vi "Add Keywords Popup Dialog.vi"(8 "error in (no error)":errorcluster, 11 "Keywords In":string[](array[string])) -> (0 "error out":errorcluster, 3 "Keywords Out":string[](array[string]))   [LabVIEW 2013, in "Intellisense Xcontrol.xctl"]
uses:
  Intellisense Xcontrol.xctl
panel:
  in  "Cancel Button":bool
  in  "OK Button":bool
  # "Enter a list of keywords"
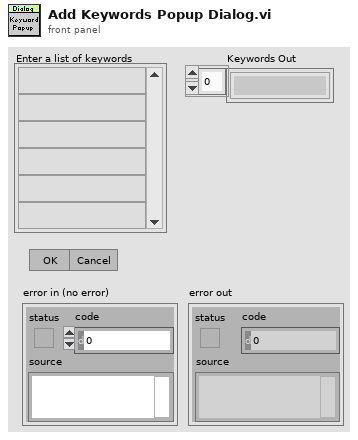
[diagram p1: front panel]
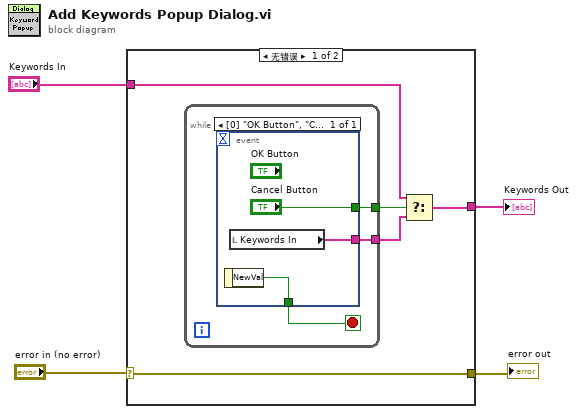
[diagram p0: block diagram]
diagram:
  n1 = case shown="无错误" "error in (no error)" {
    selector: "error in (no error)" -> [w5 w17]
    tunnel: "Keywords In" -> [w8 w16]
    tunnel: [w7 w16] -> w3
    tunnel: [w5 w17] -> w1
    frame No Error {
      n2 = while {
        tunnel: [w11] -> w9
        tunnel: [w10] -> w6
        stop <- w12 stop-if-true
        n3 = event shown="[0] \"OK Button\", \"Cancel Button\": 值改变" {
          selector: _ -> [_]
          dyn-events: _ -> [_]
          timeout: _ -> [_]
          tunnel: [w15] -> w12
          tunnel: ["Cancel Button"] -> w11
          tunnel: [w13] -> w10
          event "OK Button", "Cancel Button": Value Change {
            n4 = event-data() -> ("NewVal"=w15:bool)  [unwired: 1 in]
            n5 = local read "Keywords In"() -> (w13:string[])
          }
        }
      }
      n6 = Select(t=w8, s=w9, f=w6) -> (s? t:f=w7:string[])
    }
    frame Error {
      # "If error, do nothing."
    }
  }
  "Keywords Out" <- w3
  "error out" <- w1
